vi "Get DB info.vi"(3 "error in":errorcluster, 5 "connection reference in":T1) -> (0 "error out":errorcluster, 1 "Database Information":string[][](table), 2 "connection reference out":T1)   [LabVIEW 2010, in "SQL project lib.lvlib"]
doc: "This example returns information contained in a database named LabVIEW.mdb located in the LabVIEW examples>>database directory. The information consists of the table names, column names, data types, and data sizes."
uses:
  SQL project lib.lvlib
  <vilib>/addons/database/Connection.llb/Conn ObjectReference.ctl
  <vilib>/addons/database/NI_Database_API.lvlib
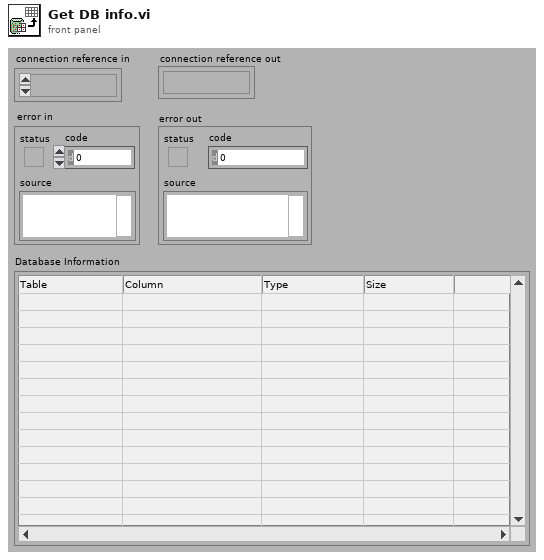
[diagram p1: front panel]
types:
  T1 = typedef "NI_Database_API.lvlib/Conn ObjectReference.ctl" = refnum<k1>
  T2 = typedef "NI_Database_API.lvlib/DB Tools DataTypes.ctl" = enum16{"String", "Long (I32)", "Single (SGL)", "Double (DBL)", "Date/Time", "Binary"}
  T3 = cluster{"name":string, "database data type":T2, "defined size":i32}[]
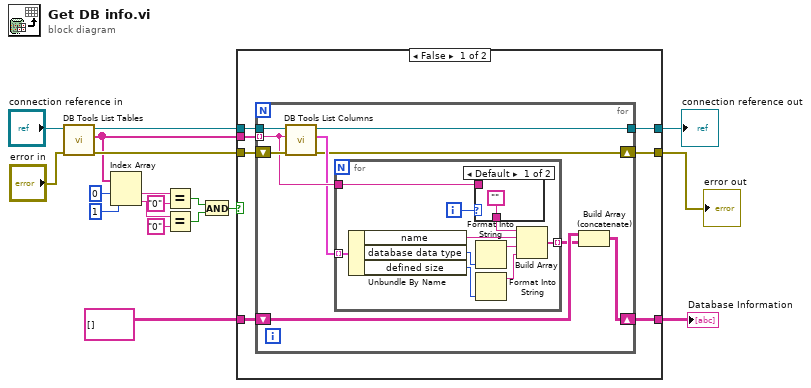
[diagram p0: block diagram]
diagram:
  n1 = call <vilib>:"DB Tools List Tables.vi"("error in (no error)"="error in", "connection reference"="connection reference in") -> ("error out"=w17:errorcluster, "tables"=w10:string[], "connection reference out"=w18:T1)  [unwired: 3 in]
  n2 = Index Array(array=w10, index #1=0 ("index"), index #2=1 ("index")) -> (element #1=w7:string, element #2=w4:string)
  n3 = Equal?(x=w7, y="0") -> (x = y?=w2:bool)
  n4 = Equal?(x=w4, y="0") -> (x = y?=w1:bool)
  n5 = And(x=w2, y=w1) -> (x .and. y?=w3:bool)
  n6 = case shown="False" w3 {
    tunnel: w18 -> [w25 w48]
    tunnel: w17 -> [w24 w47]
    tunnel: w10 -> [w23 _]
    tunnel: [w22 w49] -> w16
    tunnel: string[][] [] -> [w21 w49]
    tunnel: [w20 w47] -> w12
    tunnel: [w19 w48] -> w11
    frame False {
      n7 = for {
        tunnel: w25 -> [w33]
        shift-right: [w30] -> w20
        shift-left: w24 -> [w34]
        tunnel: w23 -> [w32] mode=indexing
        shift-right: [w29] -> w22
        shift-left: w21 -> [w28]
        tunnel: [w26] -> w19
        n8 = call <vilib>:"DB Tools List Columns.vi"("error in (no error)"=w34, "table"=w32, "connection reference"=w33) -> ("error out"=w30:errorcluster, "column information"=w31:T3, "connection reference out"=w26:T1)  [unwired: 1 in, 1 out]
        n9 = for {
          tunnel: w32 -> [w43]
          tunnel: w31 -> [w40] mode=indexing
          tunnel: [w42] -> w27 mode=indexing
          i -> [w44]
          n10 = Unbundle By Name(w40) -> ("name"=w39:string, "database data type"=w38:T2, "defined size"=w36:i32)
          n11 = case shown="Default" w44 {
            tunnel: w43 -> [_ w46]
            tunnel: ["" w46] -> w41
            frame Default {
            }
            frame 0 {
            }
          }
          n12 = Format Into String(w38) -> (resulting string=w37:string)  [unwired: 3 in, 1 out]
          n13 = Format Into String(w36) -> (resulting string=w35:string)  [unwired: 3 in, 1 out]
          n14 = Build Array(w41, w39, w37, w35) -> (w42:string[])
        }
        n15 = Build Array (concatenate)(w28, w27) -> (w29:string[][])
      }
    }
    frame True {
    }
  }
  "Database Information" <- w16
  "error out" <- w12
  "connection reference out" <- w11
